vi "Create CfgGM.vi"(8 "error in (no error)":errorcluster, 11 "Cfg Grandmaster in":refnum<class "Cfg Grandmaster.lvclass">) -> (0 "error out":errorcluster, 2 "Writer Meta data":T1[](array[typedef]), 3 "Cfg Grandmaster out":refnum<class "Cfg Grandmaster.lvclass">)   [LabVIEW 2018, in "Configuration Grandmaster.lvlib" / "Cfg Grandmaster.lvclass"]
uses:
  Cfg Grandmaster.lvclass
  <vilib>/NI/STM/compatibility/stm_MetaDataElement.ctl
  Custom Ctrls/Master Cfg/ge_Cfg wChassis.ctl
  Class Chassis BOM/Chassis BOM.lvclass
  Class Chassis Cfg/ChassisCfg.lvclass
  Data Acquisition/Class Chassis Tasks/Chassis Tasks.lvclass
  Common/Controls/TCP Ports.ctl
  Common/Controls/Selected Group.ctl
  Common/Controls/TE_Designator.ctl
  Common/Controls/Chassis Type.ctl
  Cfg Grandmaster.lvclass/Cfg Grandmaster.ctl
  <vilib>/nisyscfg/Find Hardware.vi
  <vilib>/nisyscfg/Close (System).vi
  <vilib>/nisyscfg/nisyscfg.lvlib
  <resource>/objmgr/nicontrollersysapi.rc
  <resource>/objmgr/nisysapi.rc
  <resource>/objmgr/niflexrioatomicsae.rc
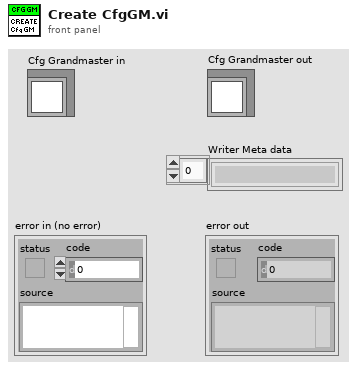
[diagram p1: front panel]
types:
  T1 = typedef "stm_MetaDataElement.ctl" = string
  T2 = typedef "Selected Group.ctl" = cluster{"ChanGroup":i32, "Rate Class":T3}
  T3 = typedef "TE_Designator.ctl" = enum16{"High Speed", "Low Speed"}
  T4 = typedef "TCP Ports.ctl" = cluster{"Port Rdr":u16, "Port HS":u16, "Port LS":u16}
  T5 = typedef "Chassis Type.ctl" = enum16{"Not Supported", "C Series 1-Slot", "C Series 4-Slot", "C Series 8-Slot", "PXI 8-Slot", "PXIe 18-Slot"}
  T6 = typedef "ge_Cfg wChassis.ctl" = cluster{"Chassis BOM":refnum<class "Chassis BOM.lvclass">, "Chassis Cfg":refnum<class "ChassisCfg.lvclass">, "Chassis Tasks":refnum<class "Chassis Tasks.lvclass">, "HW Error":bool, "Unsvd Chgs?":bool}
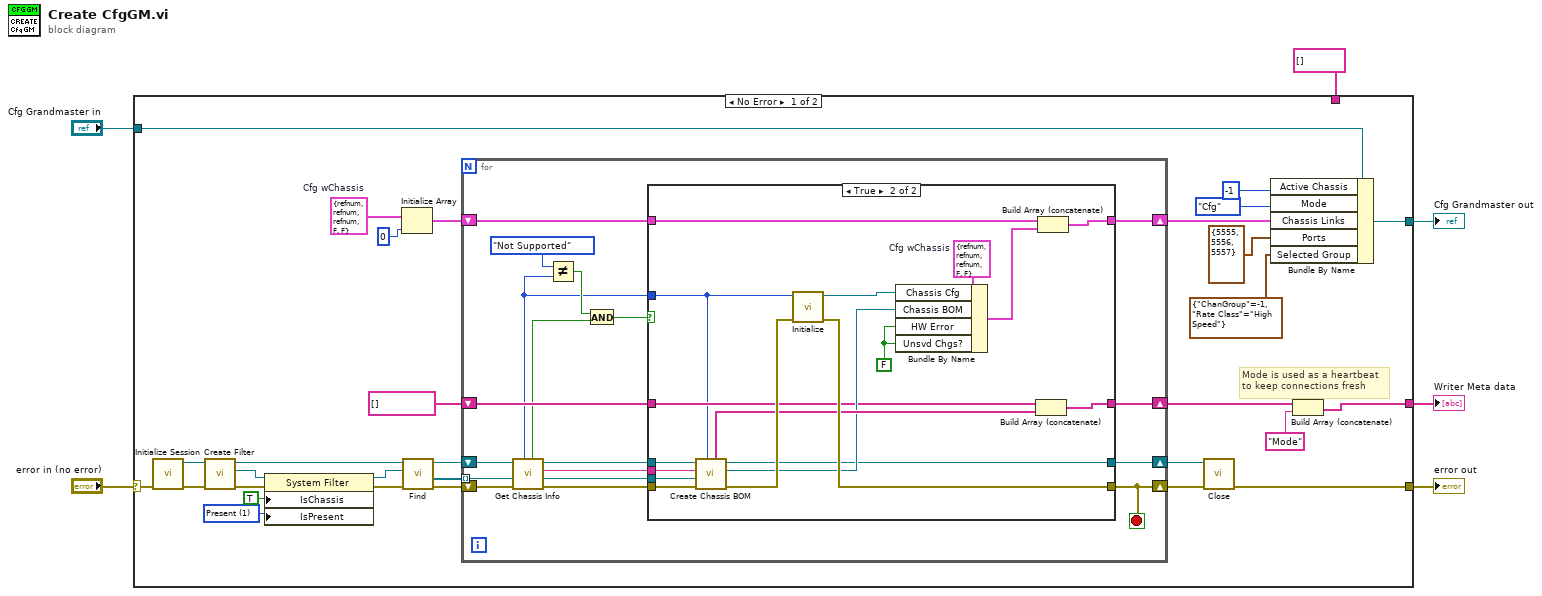
[diagram p0: block diagram]
diagram:
  n1 = case shown="No Error" "error in (no error)" {
    selector: "error in (no error)" -> [w13 w79]
    tunnel: [w23 w77] -> w6
    tunnel: [w7 w79] -> w5
    tunnel: "Cfg Grandmaster in" -> [w32 w78]
    tunnel: [w31 w78] -> w3
    tunnel: T1[] [] ("Meta data") -> [_ w77]
    frame No Error {
      w22 = 1 items=["Unknown"=-1, "Not Present"=0, "Present"=1] ("Devices & Chassis:Is Present")
      w34 = T6 {"Chassis BOM"=refnum, "Chassis Cfg"=refnum, "Chassis Tasks"=refnum, "HW Error"=FALSE, "Unsvd Chgs?"=FALSE}  # Cfg wChassis
      # "Mode is used as a heartbeat\nto keep connections fresh"
      n2 = call <vilib>:"Initialize Session.vi"("error in (no error)"=w13) -> ("error out"=w19:errorcluster, "Session out"=w16:refnum<k21>)  [unwired: 9 in]
      n3 = call <vilib>:"Create Filter.vi"("error in (no error)"=w19, "Session in"=w16) -> ("error out"=w14:errorcluster, "Filter out"=w15:refnum<k20>, "Session out"=w17:refnum<k21>)  [unwired: 7 in]
      n4 = property class="System Filter"(reference=w15, error in=w14, "IsChassis"=TRUE ("Is Chassis"), "IsPresent"=w22) -> (reference out=w21:refnum<k20>, error out=w18:errorcluster)
      n5 = Initialize Array(w34, 0 ("dimension size")) -> (w35:T6[])
      n6 = call-poly <vilib>:"Find.vi"("error in (no error)"=w18, "Filter in"=w21, "Session in"=w17) -> ("error out"=w12:errorcluster, "Resources out"=w11:refnum<k20>[], "Session out"=w10:refnum<k21>)  [unwired: 5 in, 1 out]
      n7 = for {
        shift-right: [w37] -> w8
        shift-left: w12 -> [w44]
        shift-right: [w53] -> w30
        shift-left: w35 -> [w54]
        shift-right: [w51] -> w25
        shift-left: T1[] [] ("Meta data") -> [w52]
        tunnel: w11 -> [w43] mode=indexing
        shift-right: [w41] -> w9
        shift-left: w10 -> [w50]
        stop <- w37 stop-if-true
        n8 = call "Get Chassis Info.vi"("error in"=w44, "System Hardware"=w43, "SysAPI Session"=w50) -> ("error out"=w49:errorcluster, "System Hardware"=w42:refnum<k20>, "IP Address"=w40:string, "SysAPI Session"=w45:refnum<k21>, "Device Connected?"=w38:bool, "ChassisType"=w39:T5)  [unwired: 3 in]
        n9 = Not Equal?(x=Chassis_Type."Not Supported" ("y"), y=w39) -> (x != y?=w47:bool)
        n10 = And(x=w47, y=w38) -> (x .and. y?=w46:bool)
        n11 = case shown="True" w46 {
          tunnel: w54 -> [w57 w76]
          tunnel: [w57 w75] -> w53
          tunnel: [w58 w69] -> w37
          tunnel: w45 -> [w55 w66]
          tunnel: w49 -> [w58 w68]
          tunnel: w52 -> [w56 w61]
          tunnel: [w56 w71] -> w51
          tunnel: w39 -> [_ w59]
          tunnel: w42 -> [_ w65]
          tunnel: [w55 w62] -> w41
          tunnel: w40 -> [_ w60]
          frame False {
          }
          frame True {
            w72 = FALSE ("HW Error")
            w74 = T6 {"Chassis BOM"=refnum, "Chassis Cfg"=refnum, "Chassis Tasks"=refnum, "HW Error"=FALSE, "Unsvd Chgs?"=FALSE}  # Cfg wChassis
            n12 = call "Create Chassis BOM.vi"("ChassisType"=w59, "error in (no error)"=w68, "System Hardware"=w65, "IP Addr"=w60, "SysAPI Session"=w66) -> ("error out"=w67:errorcluster, "Chassis BOM out"=w63:refnum<class "Chassis BOM.lvclass">, "SysAPI Session"=w62:refnum<k21>, "Chassis Meta Data"=w64:string[])  [unwired: 3 in]
            n13 = call "Initialize.vi"("error in"=w67, "ChassisType"=w59) -> ("error out"=w69:errorcluster, "Chassis Cfg"=w70:refnum<class "ChassisCfg.lvclass">)  [unwired: 7 in]
            n14 = Bundle By Name(cluster=w74, "Chassis Cfg"=w70, "Chassis BOM"=w63, "HW Error"=w72, "Unsvd Chgs?"=w72) -> (w73:T6)
            n15 = Build Array (concatenate)(w61, w64) -> (w71:T1[])
            n16 = Build Array (concatenate)(w76, w73) -> (w75:T6[])
          }
        }
      }
      n17 = call-poly <vilib>:"Close.vi"("error in (no error)"=w8, "Session in"=w9) -> ("error out"=w7:errorcluster)  [unwired: 9 in]
      n18 = Bundle By Name(cluster=w32, "Active Chassis"=-1, "Mode"=enum16{"Cfg", "Run"}."Cfg", "Chassis Links"=w30, "Ports"=T4 {"Port Rdr"=5555, "Port HS"=5556, "Port LS"=5557}, "Selected Group"=T2 {"ChanGroup"=-1, "Rate Class"=enum."High Speed"}) -> (w31:refnum<class "Cfg Grandmaster.lvclass">)
      n19 = Build Array (concatenate)(w25, "Mode") -> (w23:T1[])
    }
    frame Error {
    }
  }
  "Cfg Grandmaster out" <- w3
  "Writer Meta data" <- w6
  "error out" <- w5
